vi "load template description map.vi"(11 "Path":path=path "D:/github/JKI-State-Machine-Plus/.doc/VI Description.md") -> (0 "text":string, 2 "Array":string[](array[string]), 3 "variant":variant)   [LabVIEW 2014]
uses:
  JKI State Machine++.lvlib
panel:
  out "values":string
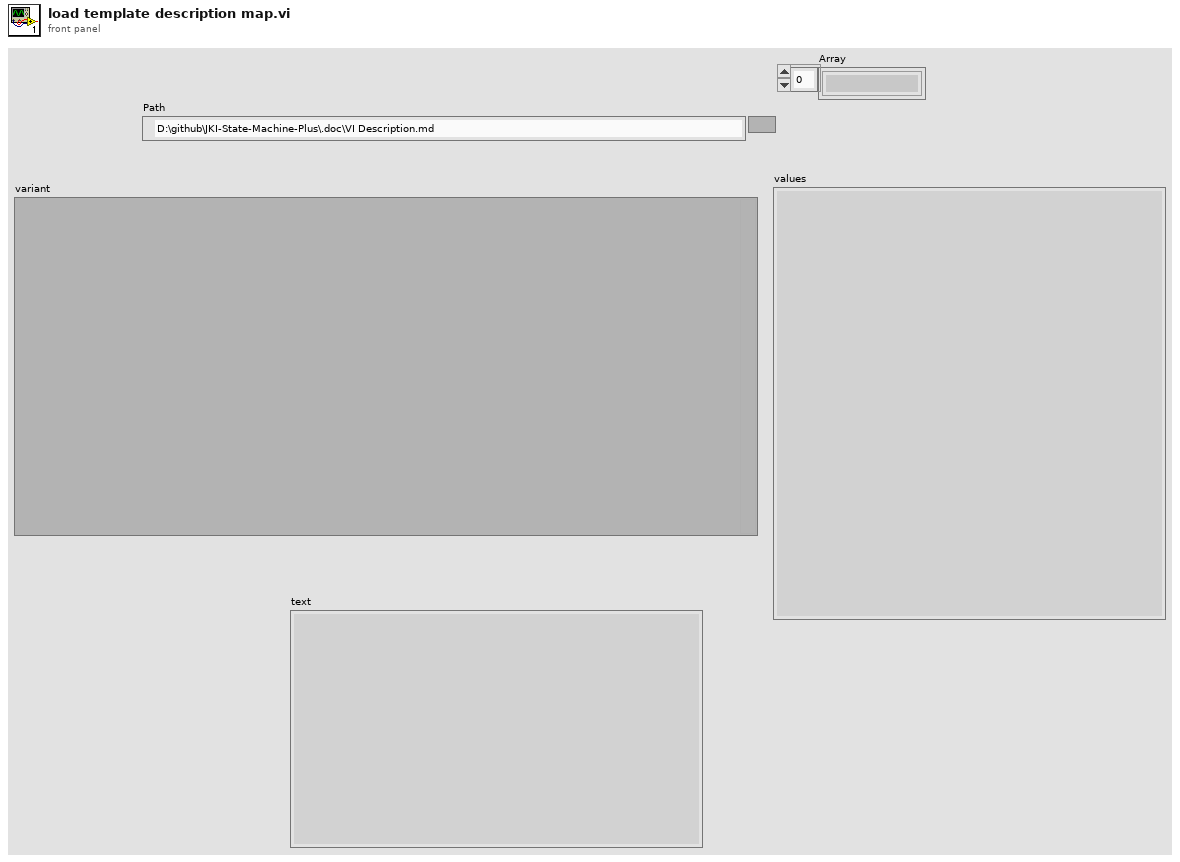
[diagram p1: front panel]
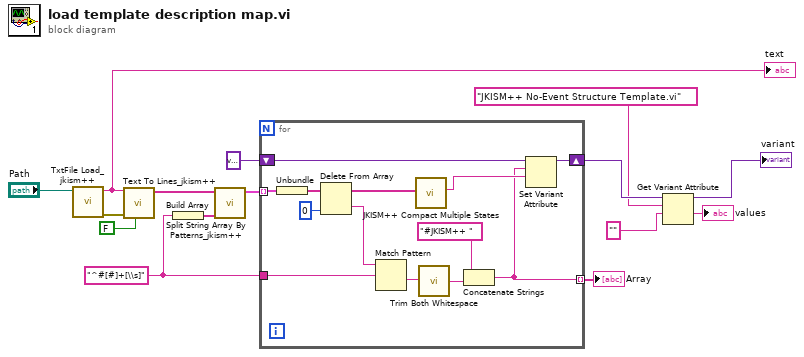
[diagram p0: block diagram]
diagram:
  w10 = "^#[#]+[\\s]" ("delimited string")
  n1 = call "TxtFile Load_jkism++.vi"("Path"="Path") -> ("error out"=w14:errorcluster, "text"=w13:string)  [unwired: 9 in]
  "text" <- w13
  n2 = call "Text To Lines_jkism++.vi"("Remove Empty Lines?(T)"=FALSE, "error in (no error)"=w14, "string"=w13) -> ("Lines"=w12:string[])  [unwired: 7 in, 1 out]
  n3 = Build Array(w10) -> (w9:string[])
  n4 = call "Split String Array By Patterns_jkism++.vi"("patterns"=w9, "Text Array"=w12) -> ("Array"=w11:cluster{"filtered array":string[]}[])  [unwired: 9 in]
  n5 = for {
    tunnel: w11 -> [w28] mode=indexing
    tunnel: w10 -> [w24]
    shift-right: [w19] -> w6
    shift-left: variant ("variant") -> [w20]
    tunnel: [w17] -> w1 mode=indexing
    n6 = Unbundle(w28) -> ("filtered array"=w27:string[])
    n7 = Delete From Array(array=w27, index=0) -> (deleted portion=w25:string, array with subset deleted=w22:string[])  [unwired: 1 in]
    n8 = Match Pattern(string=w25, regular expression=w24) -> (after substring=w23:string)  [unwired: 1 in, 3 out]
    n9 = call "JKISM++ Compact Multiple States.vi"("States in Lines"=w22) -> ("States"=w21:string)  [unwired: 9 in]
    n10 = call "Trim Both Whitespace.vi"("string"=w23) -> ("trimmed string"=w18:string)  [unwired: 1 in]
    n11 = Concatenate Strings("#JKISM++ " ("string"), w18) -> (w17:string)
    n12 = Set Variant Attribute(Variant=w20, name=w17, value=w21) -> (Variant out=w19:variant)  [unwired: 1 in, 2 out]
  }
  "Array" <- w1
  n13 = Get Variant Attribute(Variant=w6, name="JKISM++ No-Event Structure Template.vi", default value (empty Variant)="" ("delimited string")) -> (duplicate Variant=→"variant":variant, value=→"values":string)  [unwired: 1 in, 2 out]
